vi "endTriggeredLoop.vi"(8 "error in (no error)":errorcluster, 11 "Model in":refnum<class "Model.lvclass">) -> (0 "error out":errorcluster, 3 "Model out":refnum<class "Model.lvclass">)   [LabVIEW 2016, in "Model.lvclass"]
doc: "Determines the loop time (and if it is out of range) and captures a timestamp."
uses:
  Model.lvclass
  Typedefs/PubDataSV.ctl
  ts_sallv_exa/DataTypes/logevent_LoopTimeOutOfRange.ctl
  ts_sallv_exa/DataTypes/LoopTime_ms.ctl
  Model.lvclass/Model.ctl
  PubSubDataEvent/PubSubDataEvent.lvclass/PubSubDataEvent.ctl
  PubSubDataEvent/Read pubDataEvents.vi
  MiddlewareSALThisComponent/getCurrentTime.vi
  ComponentTemplateCore/ComponentModel/ComponentModelRT/LoopTimer/ILoopTimer/ILoopTimer.lvclass
  Typedefs/EXATypedefs.lvlib
  ts_sallv_exa/SALLV_EXA.lvlib
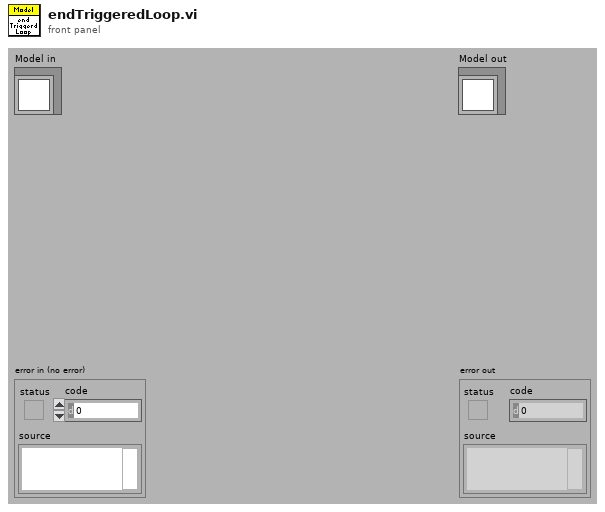
[diagram p1: front panel]
types:
  T1 = typedef "SALLV_EXA.lvlib/LoopTime_ms.ctl" = cluster{"loopTime_ms":dbl}
  T2 = typedef "SALLV_EXA.lvlib/logevent_LoopTimeOutOfRange.ctl" = cluster{"loopTimeOutOfRange":bool, "priority":i32}
  T3 = typedef "EXATypedefs.lvlib/PubDataSV.ctl" = enum16{"DetailedState", "ErrorCode", "Heartbeat", "LoopTime_ms", "LoopTimeOutOfRange", "RejectedCommand", "SummaryState", "Timestamp", "SettingVersions", "SettingsApplied", "AppliedSettingsMatchStart"}
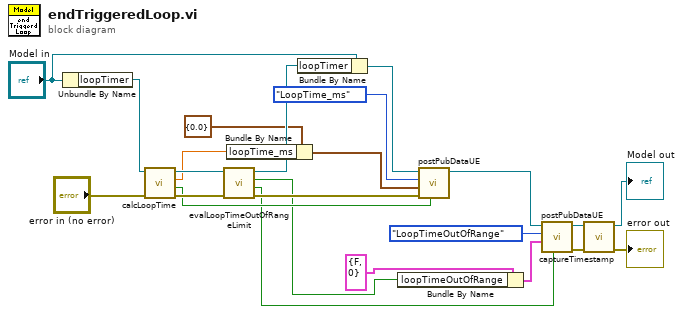
[diagram p0: block diagram]
diagram:
  n1 = Unbundle By Name("Model in") -> ("loopTimer"=w23:refnum<class "ILoopTimer.lvclass">)
  n2 = call-dynamic "calcLoopTime.vi"("error in (no error)"="error in (no error)", "ILoopTimer in"=w23) -> ("error out"=w22:errorcluster, "newValue?"=w13:bool, "loopTime_ms"=w2:dbl, "ILoopTimer out"=w21:refnum<class "ILoopTimer.lvclass">)  [unwired: 6 in]
  n3 = call-dynamic "evalLoopTimeOutOfRangeLimit.vi"("error in (no error)"=w22, "ILoopTimer in"=w21) -> ("error out"=w12:errorcluster, "newValue?"=w9:bool, "loopTimeOutOfRangeLimitActiveIsTrue"=w5:bool, "ILoopTimer out"=w19:refnum<class "ILoopTimer.lvclass">)  [unwired: 6 in]
  n4 = Bundle By Name(cluster=T1 {"loopTime_ms"=0.0} ("event data"), "loopTime_ms"=w2) -> (w1:T1)
  n5 = Bundle By Name(cluster="Model in", "loopTimer"=w19) -> (w15:refnum<class "Model.lvclass">)
  n6 = Bundle By Name(cluster=T2 {"loopTimeOutOfRange"=FALSE, "priority"=0} ("event data"), "loopTimeOutOfRange"=w5) -> (w4:T2)
  n7 = call "postPubDataUE.vi"("newValue (T)"=w13, "error in (no error)"=w12, "value"=w1, "pubDataSV"=PubDataSV."LoopTime_ms", "Model in"=w15) -> ("Model out"=w11:refnum<class "Model.lvclass">)  [unwired: 5 in, 1 out]
  n8 = call "postPubDataUE.vi"("newValue (T)"=w9, "value"=w4, "pubDataSV"=PubDataSV."LoopTimeOutOfRange", "Model in"=w11) -> ("error out"=w7:errorcluster, "Model out"=w8:refnum<class "Model.lvclass">)  [unwired: 6 in]
  n9 = call "captureTimestamp.vi"("error in (no error)"=w7, "Model in"=w8) -> ("error out"=→"error out":errorcluster, "Model out"=→"Model out":refnum<class "Model.lvclass">)  [unwired: 8 in]
